vi "BeginMeasurement.vi"(4 "error in (no error)":errorcluster, 5 "Method .NET Refnum":refnum<k24>, 6 "Live Curve Result Refnum":refnum<vi>, 7 "PalmSens in":refnum<class "PalmSens.lvclass">) -> (0 "Time Stamp":timestamp, 1 "Active Measurement Info":T1, 2 "error out":errorcluster, 3 "PalmSens out":refnum<class "PalmSens.lvclass">)   [LabVIEW 2025, in "PalmSens.lvclass"]
uses:
  PalmSens.lvclass
  E:/PSCode/PalmSens_SDK/labview/PalmSens/Libraries/PalmSens.Core.Simplified.LabVIEW.dll
  Libraries/PalmSens.Core.Simplified.LabVIEW.dll
  ActiveMeasurementInfo.ctl
  LiveCurveResult.ctl
  PalmSens.lvclass/PalmSens.ctl
panel:
  out "Method Errors":string[](array[string])
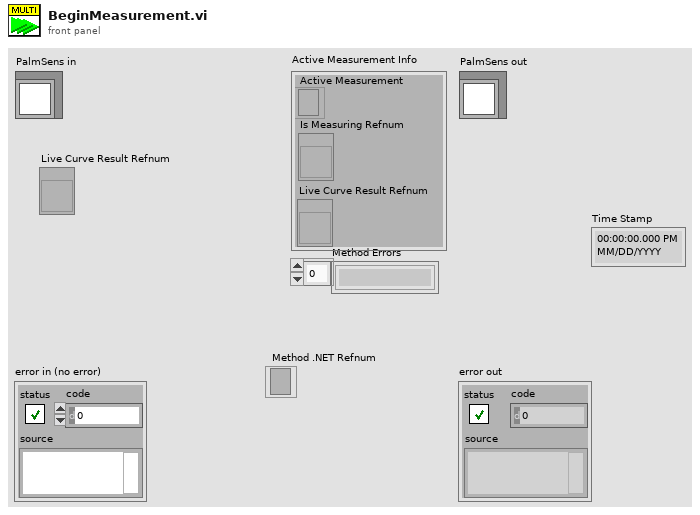
[diagram p1: front panel]
types:
  T1 = typedef "ActiveMeasurementInfo.ctl" = cluster{"Active Measurement":refnum<k24>, "Is Measuring Refnum":refnum<vi>, "Live Curve Result Refnum":refnum<vi>}
  T2 = cluster{"Active Measurement":refnum<k24>, "Is Measuring Refnum":refnum<vi>, "Live Curve Result Refnum":refnum<vi>}
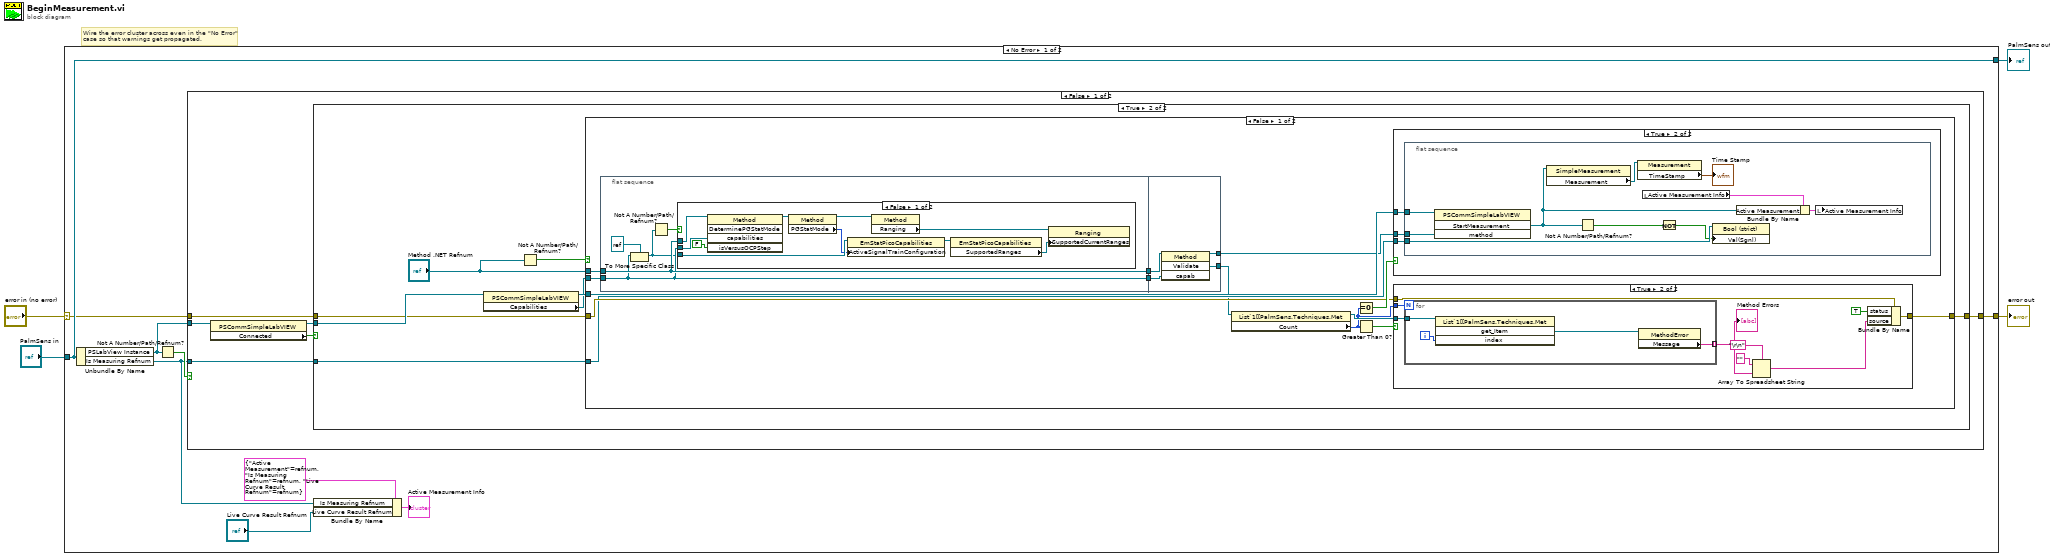
[diagram p0: block diagram]
diagram:
  # "Wire the error cluster across even in the \"No Error\"\ncase so that warnings get propagated."
  n1 = case shown="No Error" "error in (no error)" {
    selector: "error in (no error)" -> [w11 w92]
    tunnel: [w10 w92] -> w3
    tunnel: [w13 w91] -> w1
    tunnel: "PalmSens in" -> [w13 w91]
    frame No Error {
      n2 = Unbundle By Name(w13) -> ("PSLabView Instance"=w9:refnum<k24>, "Is Measuring Refnum"=w8:refnum<vi>)
      n3 = Not A Number/Path/Refnum?(number/path/refnum=w9) -> (NaN/Path/Refnum?=w12:bool)
      n4 = case shown="False" w12 {
        tunnel: w9 -> [w19 _]
        tunnel: w11 -> [w17 w90]
        tunnel: [w16 w90] -> w10
        tunnel: w8 -> [w14 _]
        frame False {
          n5 = property class="PSCommSimpleLabVIEW"(reference=w19) -> (reference out=w18:refnum<k24>, "Connected"=w15:bool)  [unwired: 1 in, 1 out]
          n6 = case shown="True" w15 {
            tunnel: [w20 w25] -> w16
            tunnel: w18 -> [_ w23]
            tunnel: w17 -> [w20 w22]
            tunnel: w14 -> [_ w21]
            frame False {
            }
            frame True {
              n7 = property class="PSCommSimpleLabVIEW"(reference=w23) -> (reference out=w27:refnum<k24>, "Capabilities"=w24:refnum<k24>)  [unwired: 1 in, 1 out]
              n8 = Not A Number/Path/Refnum?(number/path/refnum="Method .NET Refnum") -> (NaN/Path/Refnum?=w28:bool)
              n9 = case shown="False" w28 {
                tunnel: w24 -> [w42 _]
                tunnel: "Method .NET Refnum" -> [w40 _]
                tunnel: w27 -> [w39 _]
                tunnel: w22 -> [w36 w89]
                tunnel: [w35 w89] -> w25
                tunnel: w21 -> [w32 _]
                frame False {
                  n10 = flat-sequence {
                    tunnel: w40 -> [w45]
                    tunnel: w42 -> [w44]
                    tunnel: [w44] -> w34
                    tunnel: [w45] -> w33
                    tunnel: [w60] -> w31
                    tunnel: [w58] -> w38
                    tunnel: w34 -> [w61]
                    tunnel: w33 -> [w59]
                    frame #0 {
                      n11 = To More Specific Class(target class=refnum<k24> refnum, reference=w44) -> (specific class reference=w43:refnum<k24>)  [unwired: 1 in, 1 out]
                      n12 = Not A Number/Path/Refnum?(number/path/refnum=w43) -> (NaN/Path/Refnum?=w46:bool)
                      n13 = case shown="False" w46 {
                        tunnel: w45 -> [w57 _]
                        tunnel: w44 -> [w56 _]
                        tunnel: w43 -> [w55 _]
                        frame False {
                          n14 = invoke class="Method" method="DeterminePGStatMode"(reference=w57, "capabilities"=w56, "isVersusOCPStep"=FALSE) -> (reference out=w54:refnum<k24>)  [unwired: 2 in, 4 out]
                          n15 = property class="Method"(reference=w54) -> (reference out=w52:refnum<k24>, "PGStatMode"=w53:i32)  [unwired: 1 in, 1 out]
                          n16 = property class="EmStatPicoCapabilities"(reference=w55, "ActiveSignalTrainConfiguration"=w53) -> (reference out=w50:refnum<k24>)  [unwired: 1 in, 1 out]
                          n17 = property class="Method"(reference=w52) -> ("Ranging"=w51:refnum<k24>)  [unwired: 1 in, 2 out]
                          n18 = property class="EmStatPicoCapabilities"(reference=w50) -> ("SupportedRanges"=w48:refnum<k24>)  [unwired: 1 in, 2 out]
                          n19 = property class="Ranging"(reference=w51, "SupportedCurrentRanges"=w48) -> ()  [unwired: 1 in, 2 out]
                        }
                        frame True {
                        }
                      }
                    }
                    frame #1 {
                      n20 = invoke class="Method" method="Validate"(reference=w59, "capab"=w61) -> (reference out=w58:refnum<k24>, "Validate"=w60:refnum<k24>)  [unwired: 2 in, 2 out]
                    }
                  }
                  n21 = property class="List`1[[PalmSens.Techniques.Met"(reference=w31) -> (reference out=w30:refnum<k24>, "Count"=w29:i32)  [unwired: 1 in, 1 out]
                  n22 = Equal To 0?(x=w29) -> (x = 0?=w41:bool)
                  n23 = Greater Than 0?(x=w29) -> (x > 0?=w37:bool)
                  n24 = case shown="True" w41 {
                    tunnel: w39 -> [_ w78]
                    tunnel: w38 -> [_ w77]
                    tunnel: w32 -> [_ w76]
                    frame False {
                    }
                    frame True {
                      n25 = flat-sequence {
                        tunnel: w78 -> [w88]
                        tunnel: w77 -> [w87]
                        tunnel: w76 -> [w84]
                        frame #0 {
                          n26 = invoke class="PSCommSimpleLabVIEW" method="StartMeasurement"(reference=w88, "method"=w87) -> ("StartMeasurement"=w81:refnum<k24>)  [unwired: 2 in, 3 out]
                          n27 = property class="SimpleMeasurement"(reference=w81) -> ("Measurement"=w79:refnum<k24>)  [unwired: 1 in, 2 out]
                          n28 = Not A Number/Path/Refnum?(number/path/refnum=w81) -> (NaN/Path/Refnum?=w83:bool)
                          n29 = property class="Measurement"(reference=w79) -> ("TimeStamp"=→"Time Stamp":timestamp)  [unwired: 1 in, 2 out]
                          n30 = local read "Active Measurement Info"() -> (w86:T1)
                          n31 = Not(x=w83) -> (.not. x?=w82:bool)
                          n32 = property class="Bool (strict)"(reference=w84, "Val(Sgnl)"=w82) -> ()  [unwired: 1 in, 2 out]
                          n33 = Bundle By Name(cluster=w86, "Active Measurement"=w81) -> (w85:T1)
                          n34 = local write "Active Measurement Info"(w85) -> ()
                        }
                      }
                    }
                  }
                  n35 = case shown="True" w37 {
                    tunnel: w29 -> [_ w71]
                    tunnel: w30 -> [_ w70]
                    tunnel: w36 -> [w62 w69]
                    tunnel: [w62 w68] -> w35
                    frame False {
                    }
                    frame True {
                      n36 = for {
                        N: w71 -> [_]
                        tunnel: [w75] -> w63 mode=indexing
                        tunnel: w70 -> [w74]
                        i -> [w73]
                        n37 = invoke class="List`1[[PalmSens.Techniques.Met" method="get_Item"(reference=w74, "index"=w73) -> ("get_Item"=w72:refnum<k24>)  [unwired: 2 in, 3 out]
                        n38 = property class="MethodError"(reference=w72) -> ("Message"=w75:string)  [unwired: 1 in, 2 out]
                      }
                      "Method Errors" <- w63
                      n39 = Array To Spreadsheet String(delimiter (Tab)="\r\n", array=w63, 3:"" ("format string")) -> (spreadsheet string=w66:string)
                      n40 = Bundle By Name(cluster=w69, "status"=TRUE, "source"=w66) -> (w68:errorcluster)
                    }
                  }
                }
                frame True {
                }
              }
            }
          }
        }
        frame True {
        }
      }
      n41 = Bundle By Name(cluster=T2 {"Active Measurement"=refnum, "Is Measuring Refnum"=refnum, "Live Curve Result Refnum"=refnum} ("Active Measurement Info"), "Is Measuring Refnum"=w8, "Live Curve Result Refnum"="Live Curve Result Refnum") -> (→"Active Measurement Info":T2)
    }
    frame Error {
    }
  }
  "error out" <- w3
  "PalmSens out" <- w1
